vi "2D_to_1D_array.vi"(5 "2D Array in":dbl[][](array[numeric])) -> (2 "1D Array out":dbl[](array[numeric]))   [LabVIEW 2017]
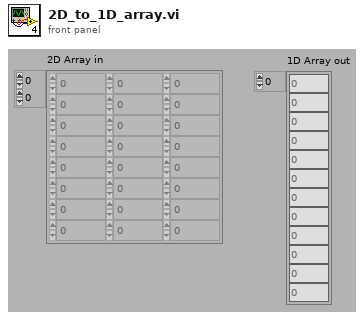
[diagram p1: front panel]
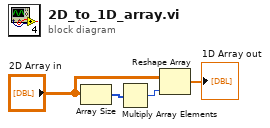
[diagram p0: block diagram]
diagram:
  n1 = Array Size(array="2D Array in") -> (size(s)=w4:i32[])
  n2 = Multiply Array Elements(1:w4) -> (0:w3:i32)
  n3 = Reshape Array("2D Array in", w3) -> (→"1D Array out":dbl[])
